vi "Post4ChartImages.vi"(6 "URL":string, 7 "Experiment Identifier":string, 8 "Transconductance..":refnum<vi>, 9 "Transconductance":refnum<vi>, 10 "Conductance..":refnum<vi>, 11 "Conductance":refnum<vi>) -> ()   [LabVIEW 2016]
panel:
  out "error out 5":errorcluster
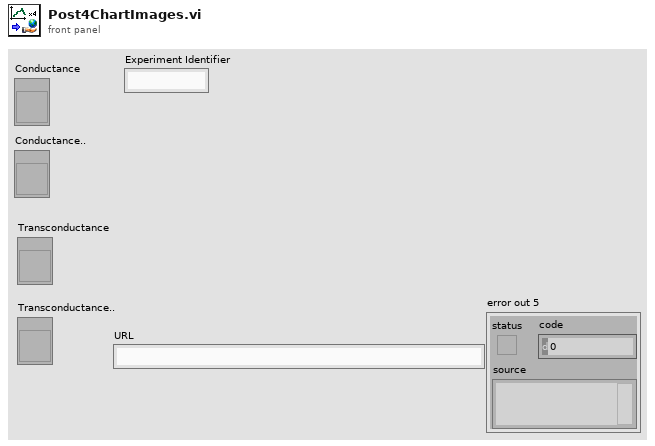
[diagram p1: front panel]
types:
  T1 = cluster{"name or relative path":string, "name or relative path 2":string, "name or relative path 3":string, "name or relative path 4":string}
  T2 = typedef "imagedata.ctl" = cluster{"image type":i32, "image depth":i32, "image":u8[], "mask":u8[], "colors":u32[], "Rectangle":cluster{"left":i16, "top":i16, "right":i16, "bottom":i16}}
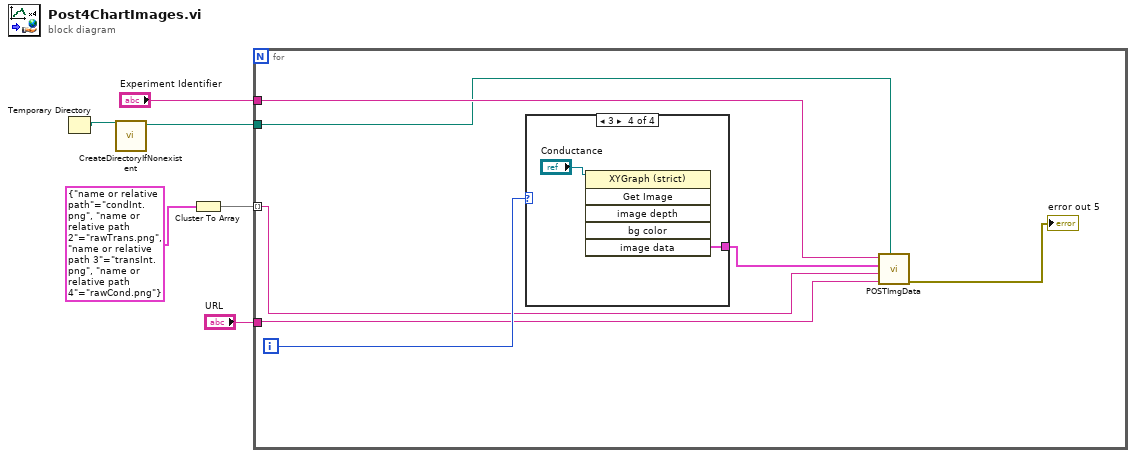
[diagram p0: block diagram]
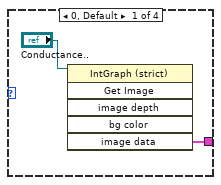
[diagram p2: hidden frame]
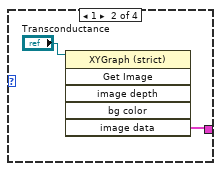
[diagram p3: hidden frame]
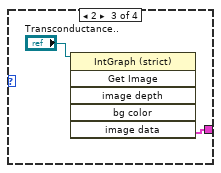
[diagram p4: hidden frame]
diagram:
  n1 = Temporary Directory() -> (w6:path)
  n2 = call "CreateDirectoryIfNonexistent.vi"("selected path"=w6) -> ("path"=w5:path)  [unwired: 10 in]
  n3 = Cluster To Array(cluster=T1 {"name or relative path"="condInt.png", "name or relative path 2"="rawTrans.png", "name or relative path 3"="transInt.png", "name or relative path 4"="rawCond.png"}) -> (array=w2:string[])
  n4 = for {
    tunnel: w5 -> [w7]
    tunnel: "Experiment Identifier" -> [w8]
    tunnel: w2 -> [w10] mode=indexing
    tunnel: "URL" -> [w9]
    i -> [w13]
    n5 = case shown="3" w13 {
      tunnel: [w15 w17 w19 w21] -> w12
      frame 0, Default {
        n6 = invoke class="IntGraph (strict)" method="Get Image"(reference="Conductance..") -> ("image data"=w15:T2)  [unwired: 5 in, 5 out]
      }
      frame 1 {
        n7 = invoke class="XYGraph (strict)" method="Get Image"(reference="Transconductance") -> ("image data"=w17:T2)  [unwired: 5 in, 5 out]
      }
      frame 2 {
        n8 = invoke class="IntGraph (strict)" method="Get Image"(reference="Transconductance..") -> ("image data"=w19:T2)  [unwired: 5 in, 5 out]
      }
      frame 3 {
        n9 = invoke class="XYGraph (strict)" method="Get Image"(reference="Conductance") -> ("image data"=w21:T2)  [unwired: 5 in, 5 out]
      }
    }
    n10 = call "POSTImgData.vi"("base path"=w7, "URL"=w9, "name or relative path"=w10, "image data"=w12, "unique experiment identifier"=w8) -> ("error out"=→"error out 5":errorcluster)  [unwired: 6 in]
  }
